vi "Pump Status.vi"(8 "error in (no error)":errorcluster, 11 "KNF Settings":T2={"VISA resource name"="", "Simulated?"=TRUE}) -> (0 "error out":errorcluster, 1 "Connection Error":bool, 2 "Pump On?":enum16{"Off", "On", "Not Initialized"}(ring), 3 "KNF Settings":T2={"VISA resource name"="", "Simulated?"=TRUE})   [LabVIEW 2018, in "KNF SIMDOS.lvlib"]
uses:
  KNF SIMDOS.lvlib
  Settings Cluster plus SIMDOS.ctl
  <vilib>/KNF LAB/Driver S/Lvlib/SIMLAB_driver_lvclass/StatusRequestMode.ctl
  <vilib>/KNF LAB/Driver S/Lvlib/SIMLAB_driver_lvclass/SIMLAB_driver.lvclass
panel:
  out "PumpStatus":T1 caption="Pump Status"
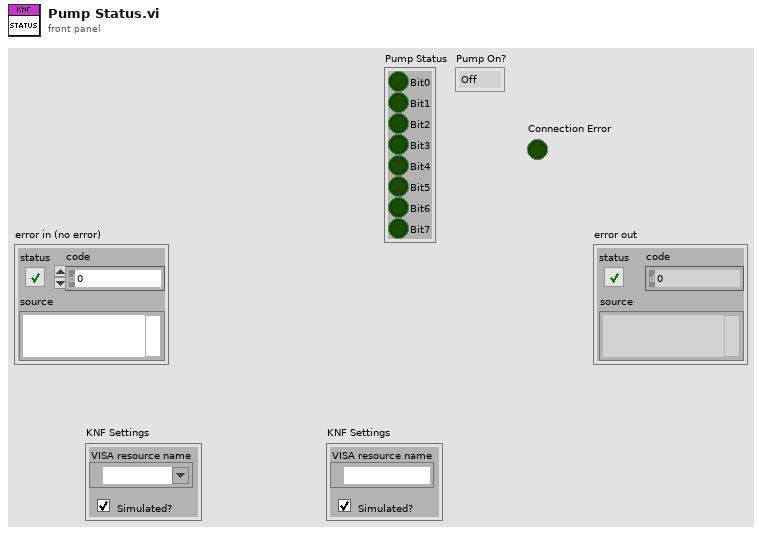
[diagram p1: front panel]
types:
  T1 = cluster{"Bit0":bool, "Bit1":bool, "Bit2":bool, "Bit3":bool, "Bit4":bool, "Bit5":bool, "Bit6":bool, "Bit7":bool}
  T2 = typedef "KNF SIMDOS.lvlib/Settings Cluster plus SIMDOS.ctl" = cluster{"VISA resource name":refnum<visa-resource-name>, "Simulated?":bool}
  T3 = typedef "SIMLAB_driver.lvlib/SIMLAB_driver.lvclass/StatusRequestMode.ctl" = u16
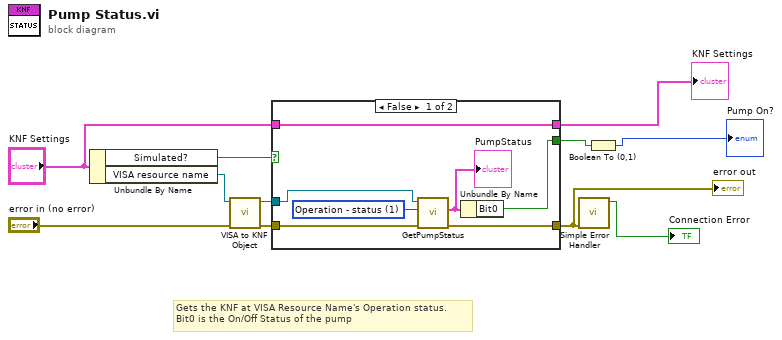
[diagram p0: block diagram]
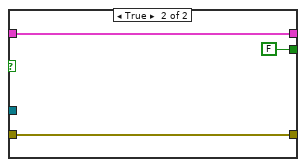
[diagram p2: hidden frame]
diagram:
  # "Gets the KNF at VISA Resource Name's Operation status.\nBit0 is the On/Off Status of the pump"
  n1 = Unbundle By Name("KNF Settings") -> ("Simulated?"=w11:bool, "VISA resource name"=w3:refnum<visa-resource-name>)
  n2 = call "VISA to KNF Object.vi"("error in (no error)"="error in (no error)", "VISA resource name"=w3) -> ("error out"=w5:errorcluster, "SIMDOS out"=w4:refnum<class "SIMLAB_driver.lvclass">)  [unwired: 8 in]
  n3 = case shown="False" w11 {
    tunnel: [w12 w21] -> w10
    tunnel: "KNF Settings" -> [w12 w21]
    tunnel: [w15 w20] -> w8
    tunnel: w5 -> [w14 w20]
    tunnel: w4 -> [w13 _]
    tunnel: [w16 FALSE] -> w2
    frame False {
      w18 = T3 1 items=["Operation - status"=1, "System - status"=2, "Run mode - status"=3, "Dispense mode - status"=4, "Reserved"=5, "Fault diagnosis"=6] ("StatusRequestMode")
      n4 = call <vilib>:"GetPumpStatus.vi"("error in (no error)"=w14, "StatusRequestMode"=w18, "SIMDOS in"=w13) -> ("error out"=w15:errorcluster, "PumpStatus"=w17:T1)  [unwired: 6 in, 1 out]
      "PumpStatus" <- w17
      n5 = Unbundle By Name(w17) -> ("Bit0"=w16:bool)
    }
    frame True {
    }
  }
  "error out" <- w8
  "KNF Settings" <- w10
  n6 = call <vilib>:"Simple Error Handler.vi"("error in (no error)"=w8) -> ("error?"=→"Connection Error":bool)  [unwired: 4 in, 4 out]
  n7 = Boolean To (0,1)(Boolean=w2) -> (0, 1=→"Pump On?":i16)
